vi "MIC_coMD.vi"() -> ()   [LabVIEW 2012]
doc: "SciScan 1.2 160622"
uses:
  GFG/GFGfpRefGet.vi
  GFG/GFGnumericGet.vi
  GFG/GFG library.lvlib
panel:
  out "Source VI":string
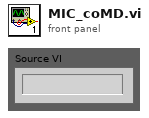
[diagram p1: front panel]
types:
  T1 = enum8{"Enabled", "Disabled", "Disabled and Grayed Out"}
  T2 = cluster{"WaveformChartRef":refnum<vi>, "DigitalRef":refnum<vi>, "ArrayRef":refnum<vi>, "TabControlRef":refnum<vi>, "EnumRef":refnum<vi>, "RingRef":refnum<vi>, "BooleanRef":refnum<vi>, "KnobRef":refnum<vi>, "SlideRef":refnum<vi>, "PathRef":refnum<vi>, "StringRef":refnum<vi>, "ComboBox":refnum<vi>, "WaveformGraphRef":refnum<vi>}
  T3 = enum16{"Left Button", "Center Button", "Right Button", "Window Close"}
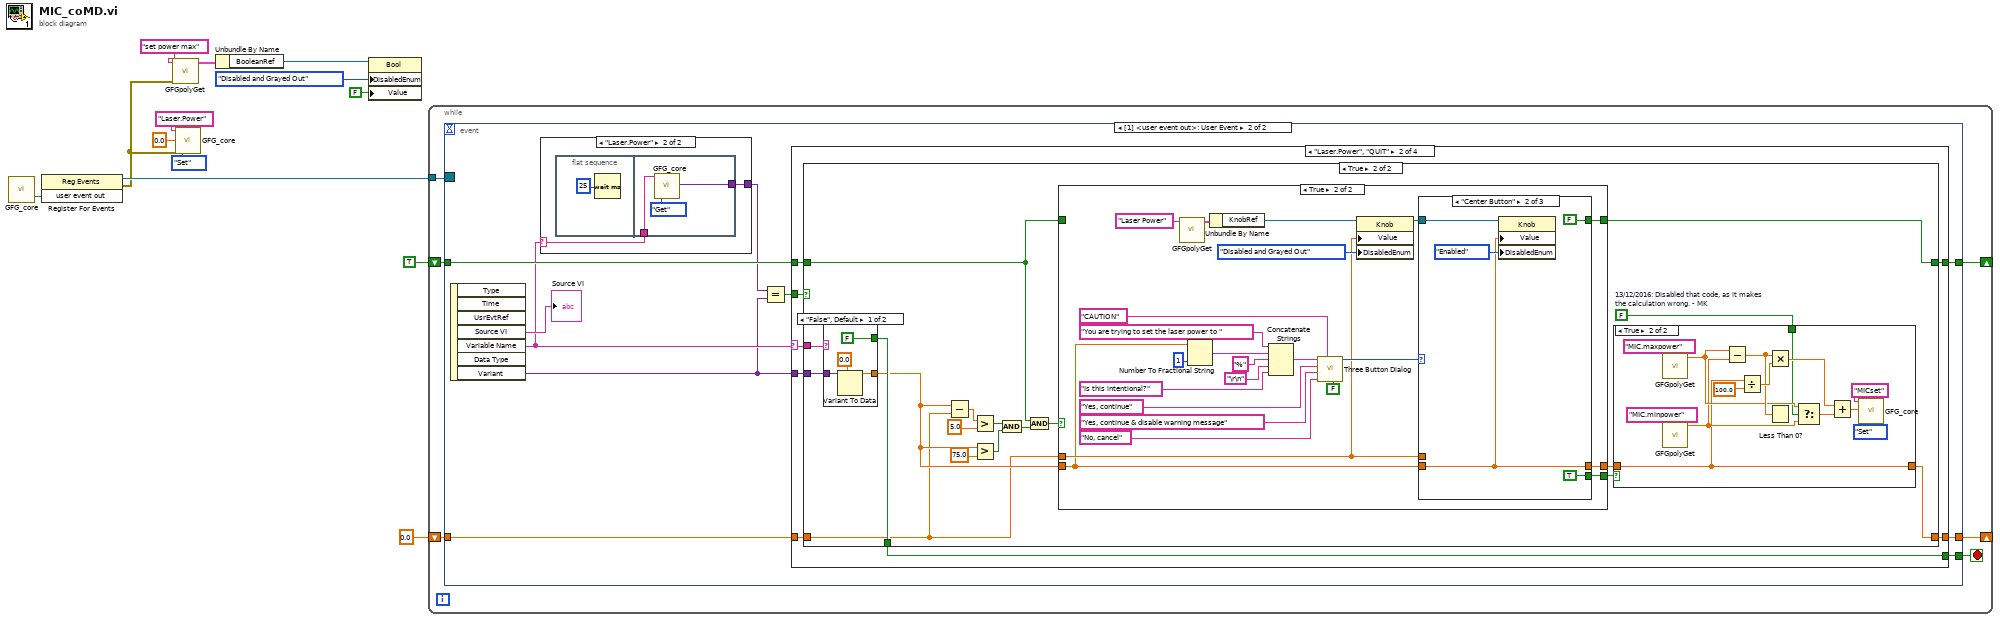
[diagram p0: block diagram]
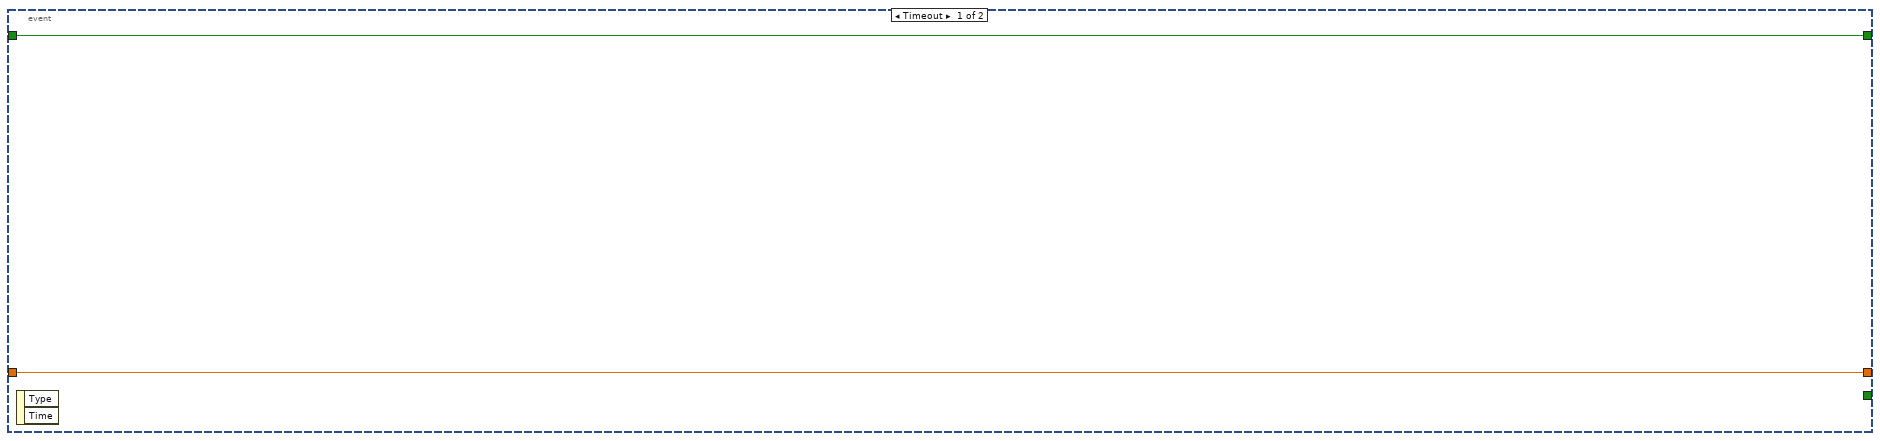
[diagram p2: hidden frame]
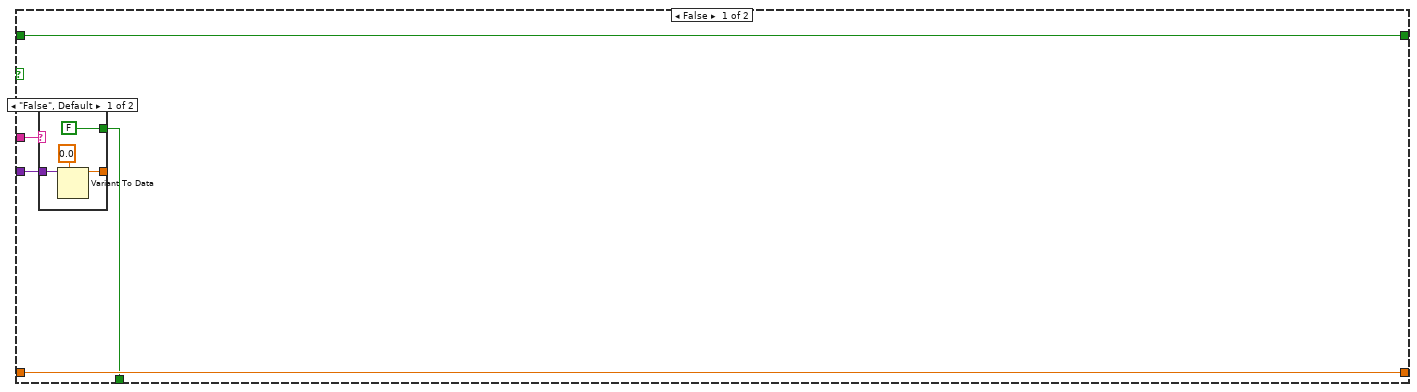
[diagram p5: hidden frame]
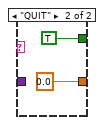
[diagram p6: hidden frame]
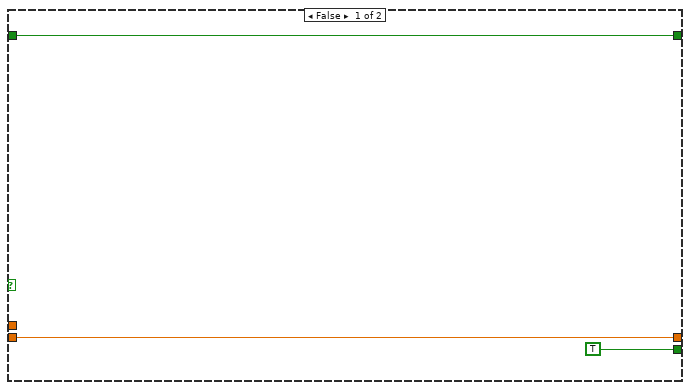
[diagram p8: hidden frame]
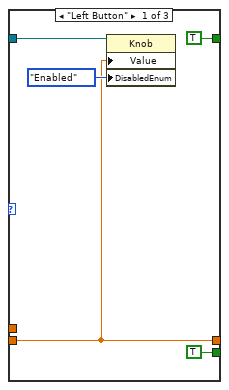
[diagram p9: hidden frame]
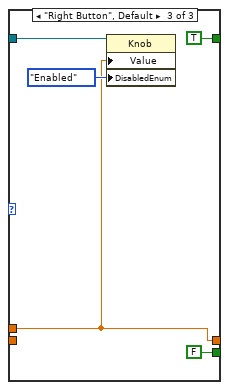
[diagram p10: hidden frame]
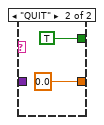
[diagram p11: hidden frame]
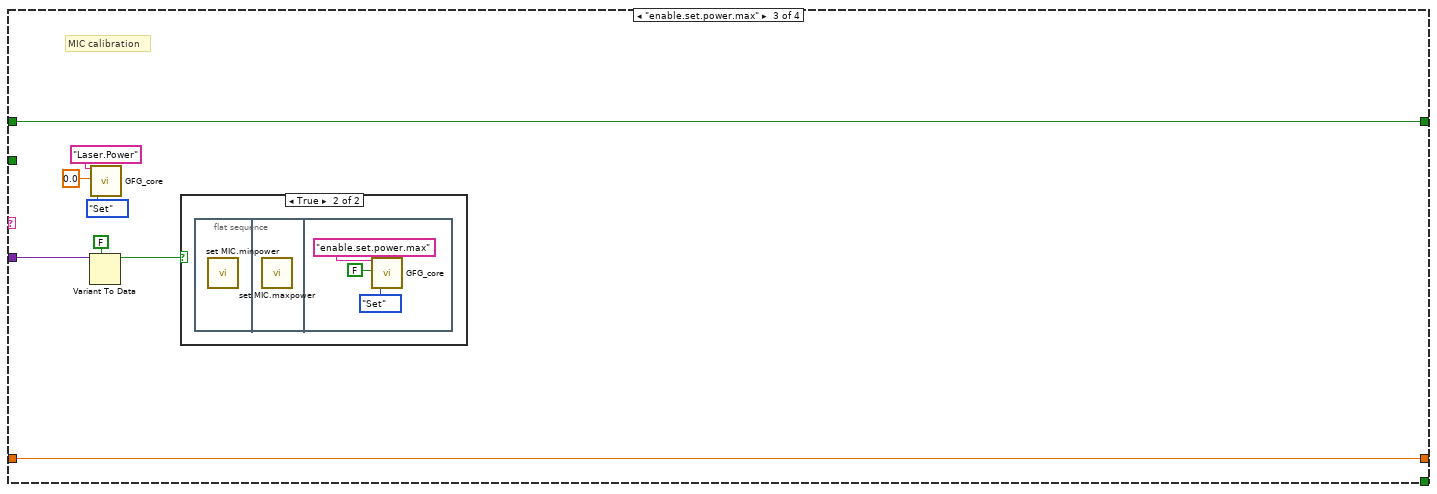
[diagram p12: hidden frame]
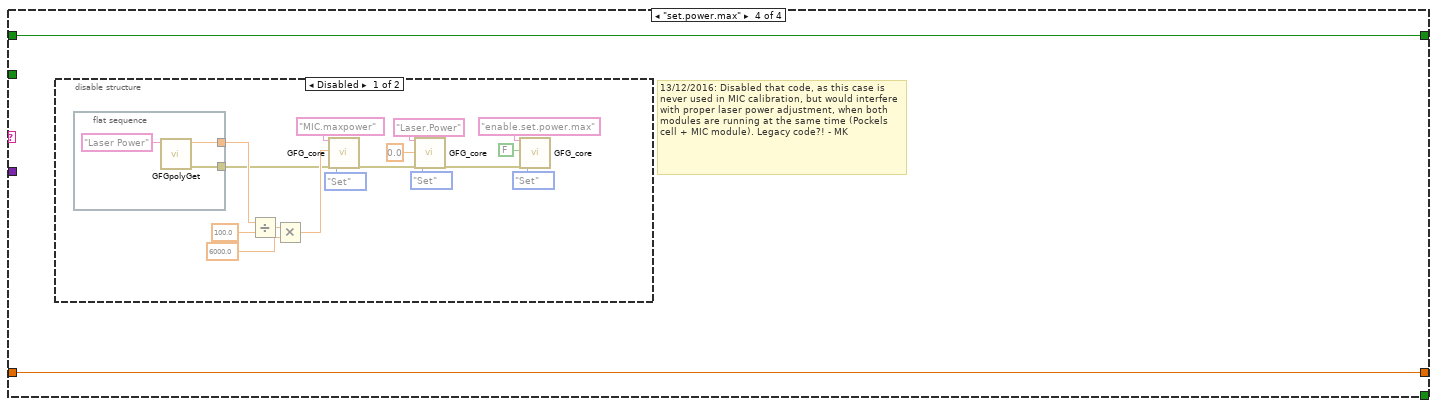
[diagram p14: hidden frame]
diagram:
  n1 = call "GFG_core.vi"() -> ("user event out"=w13:refnum<user-event>)  [unwired: 13 in, 6 out]
  n2 = register-events(w13) -> (reference out=w12:refnum<event-registration>, error out=w1:errorcluster)  [unwired: 2 in]
  n3 = call-poly "GFGpolyGet.vi"("error in (no error)"=w1, "Variable Name in"="set power max") -> ("output cluster"=w4:T2)  [unwired: 8 in, 1 out]
  n4 = call "GFG_core.vi"("Variable Name in"="Laser.Power", "Variant in"=0.0 ("Laser Power"), "error in (no error)"=w1, "Action"=enum16{"Init", "Set", "Get"}."Set") -> ()  [unwired: 9 in, 7 out]
  n5 = Unbundle By Name(w4) -> ("BooleanRef"=w5:refnum<vi>)
  n6 = property class="Bool"(reference=w5, "DisabledEnum"=T1."Disabled and Grayed Out" ("Disabled"), "Value"=FALSE) -> ()  [unwired: 1 in, 2 out]
  n7 = while {
    tunnel: w12 -> [w19]
    shift-right: [w17] -> _
    shift-left: 0.0 ("Laser Power") -> [w16]
    shift-right: [w15] -> _
    shift-left: TRUE -> [w14]
    stop <- w18 stop-if-true
    n8 = event shown="[1] <user event out>: User Event" {
      selector: w19 -> [_ _]
      dyn-events: _ -> [_ _]
      timeout: _ -> [_ _]
      tunnel: [_ w30] -> w18
      tunnel: [w21 w29] -> w17
      tunnel: w16 -> [w21 w28]
      tunnel: [w20 w27] -> w15
      tunnel: w14 -> [w20 w26]
      event Timeout {
        n9 = event-data() -> ()  [unwired: 1 in, 2 out]
      }
      event User Event {
        n10 = event-data() -> ("Source VI"=→"Source VI":string, "Variable Name"=w23:string, "Variant"=w22:variant)  [unwired: 1 in, 4 out]
        n11 = case shown="\"Laser.Power\"" w23 {
          selector: w23 -> [w32 w33]
          tunnel: [w32 w34] -> w25
          frame "False", Default {
          }
          frame "Laser.Power" {
            n12 = flat-sequence {
              tunnel: w33 -> [w37]
              tunnel: [w36] -> w34
              frame #0 {
                n13 = Wait (ms)(milliseconds to wait=u32 25) -> ()  [unwired: 1 out]
              }
              frame #1 {
                n14 = call "GFG_core.vi"("Variable Name in"=w37, "Action"=enum16{"Init", "Set", "Get"}."Get") -> ("Variant Out"=w36:variant)  [unwired: 11 in, 6 out]
              }
            }
          }
        }
        n15 = Equal?(x=w25, y=w22) -> (x = y?=w24:bool)
        n16 = case shown="\"Laser.Power\", \"QUIT\"" w23 {
          selector: w23 -> [_ w47 _ _]
          tunnel: w22 -> [_ w48 w142 _]
          tunnel: [_ w46 _ _] -> w30
          tunnel: [w40 w43 w147 w152] -> w29
          tunnel: w28 -> [w40 w42 w147 w152]
          tunnel: [w39 w45 w146 w151] -> w27
          tunnel: w26 -> [w39 w44 w146 w151]
          tunnel: w24 -> [_ w41 _ _]
          frame Default {
          }
          frame "Laser.Power", "QUIT" {
            n17 = case shown="True" w41 {
              tunnel: w48 -> [w51 w77]
              tunnel: w47 -> [w50 w76]
              tunnel: [w49 w75] -> w46
              tunnel: [w52 w72] -> w45
              tunnel: w44 -> [w52 w70]
              tunnel: [w53 w61] -> w43
              tunnel: w42 -> [w53 w66]
              frame False {
                n18 = case shown="\"False\", Default" w50 {
                  tunnel: w51 -> [w57 _]
                  tunnel: [w56 0.0 ("Laser Power")] -> _
                  tunnel: [FALSE TRUE] -> w49
                  frame "False", Default {
                    n19 = Variant To Data(type=0.0 ("Laser Power"), Variant=w57) -> (data=w56:dbl)  [unwired: 1 in, 1 out]
                  }
                  frame "QUIT" {
                  }
                }
              }
              frame True {
                w60 = FALSE  # 13/12/2016: Disabled that code, as it makes the calculation wrong. - MK
                n20 = case shown="\"False\", Default" w76 {
                  tunnel: w77 -> [w137 _]
                  tunnel: [w136 0.0 ("Laser Power")] -> w67
                  tunnel: [FALSE TRUE] -> w75
                  frame "False", Default {
                    n21 = Variant To Data(type=0.0 ("Laser Power"), Variant=w137) -> (data=w136:dbl)  [unwired: 1 in, 1 out]
                  }
                  frame "QUIT" {
                  }
                }
                n22 = Subtract(x=w67, y=w66) -> (x-y=w65:dbl)
                n23 = Greater?(x=w65, y=5.0) -> (0:w63:bool)
                n24 = Greater?(x=w67, y=75.0) -> (0:w74:bool)
                n25 = And(x=w63, y=w74) -> (x .and. y?=w68:bool)
                n26 = And(x=w70, y=w68) -> (x .and. y?=w71:bool)
                n27 = case shown="True" w71 {
                  tunnel: [TRUE w112] -> w62
                  tunnel: [w94 w111] -> w72
                  tunnel: w70 -> [w94 _]
                  tunnel: w66 -> [_ w101]
                  tunnel: w67 -> [w93 w96]
                  tunnel: [w93 w97] -> w69
                  frame False {
                  }
                  frame True {
                    n28 = call-poly "GFGpolyGet.vi"("Variable Name in"="Laser Power") -> ("output cluster"=w105:T2)  [unwired: 9 in, 1 out]
                    n29 = Number To Fractional String(number=w96, precision (6)=i16 1) -> (F-format string=w100:string)  [unwired: 2 in]
                    n30 = Unbundle By Name(w105) -> ("KnobRef"=w104:refnum<vi>)
                    n31 = Concatenate Strings("You are trying to set the laser power to " ("message"), w100, "%" ("string"), "\r\n", "Is this intentional?" ("string")) -> (w107:string)
                    n32 = call <vilib>:"Three Button Dialog.vi"("Allow user to close window? (TRUE)"=FALSE, "Window Title (\"\")"="CAUTION" ("Window Title (\"\")"), "Right Button Text (\"Cancel\")"="No, cancel" ("Right Button Text (\"Cancel\")"), "Center Button Text (\"No\")"="Yes, continue & disable warning message" ("Center Button Text (\"No\")"), "Left Button Text (\"Yes\")"="Yes, continue" ("Left Button Text (\"Yes\")"), "message"=w107) -> ("Which Button?"=w113:T3)  [unwired: 5 in]
                    n33 = property class="Knob"(reference=w104, "Value"=w101, "DisabledEnum"=T1."Disabled and Grayed Out" ("Disabled")) -> (reference out=w102:refnum<vi>)  [unwired: 1 in, 1 out]
                    n34 = case shown="\"Center Button\"" w113 {
                      tunnel: [TRUE TRUE FALSE] -> w112
                      tunnel: [TRUE FALSE TRUE] -> w111
                      tunnel: w102 -> [w120 w125 w130]
                      tunnel: w96 -> [w119 w124 _]
                      tunnel: w101 -> [_ _ w129]
                      tunnel: [w119 w124 w129] -> w97
                      frame "Left Button" {
                        n35 = property class="Knob"(reference=w120, "Value"=w119, "DisabledEnum"=T1."Enabled" ("Disabled")) -> ()  [unwired: 1 in, 2 out]
                      }
                      frame "Center Button" {
                        n36 = property class="Knob"(reference=w125, "Value"=w124, "DisabledEnum"=T1."Enabled" ("Disabled")) -> ()  [unwired: 1 in, 2 out]
                      }
                      frame "Right Button", Default {
                        n37 = property class="Knob"(reference=w130, "Value"=w129, "DisabledEnum"=T1."Enabled" ("Disabled")) -> ()  [unwired: 1 in, 2 out]
                      }
                    }
                  }
                }
                n38 = case shown="True" w62 {
                  tunnel: w69 -> [w78 w80]
                  tunnel: [w78 w80] -> w61
                  tunnel: w60 -> [_ w79]
                  frame False {
                  }
                  frame True {
                    n39 = call-poly "GFGpolyGet.vi"("Variable Name in"="MIC.maxpower") -> ("Numeric"=w86:dbl)  [unwired: 8 in, 2 out]
                    n40 = call-poly "GFGpolyGet.vi"("Variable Name in"="MIC.minpower") -> ("Numeric"=w83:dbl)  [unwired: 8 in, 2 out]
                    n41 = Subtract(x=w86, y=w83) -> (x-y=w87:dbl)
                    n42 = Divide(x=w80, y=100.0 ("x")) -> (x/y=w92:dbl)
                    n43 = Multiply(x=w87, y=w92) -> (x*y=w90:dbl)
                    n44 = Less Than 0?(x=w87) -> ()  [unwired: 1 out]
                    n45 = Select(t=w86, s=w79, f=w83) -> (s? t:f=w84:dbl)
                    n46 = Add(x=w90, y=w84) -> (x+y=w85:dbl)
                    n47 = call "GFG_core.vi"("Variable Name in"="MICset", "Variant in"=w85, "Action"=enum16{"Init", "Set", "Get"}."Set") -> ()  [unwired: 10 in, 7 out]
                  }
                }
              }
            }
          }
          frame "enable.set.power.max" {
            # "MIC calibration"
            n48 = Variant To Data(type=FALSE, Variant=w142) -> (data=w140:bool)  [unwired: 1 in, 1 out]
            n49 = call "GFG_core.vi"("Variable Name in"="Laser.Power", "Variant in"=0.0 ("Laser Power"), "Action"=enum16{"Init", "Set", "Get"}."Set") -> ()  [unwired: 10 in, 7 out]
            n50 = case shown="True" w140 {
              frame False {
              }
              frame True {
                n51 = flat-sequence {
                  frame #0 {
                    n52 = call "set MIC.minpower.vi"() -> ()  [unwired: 12 in]
                  }
                  frame #1 {
                    n53 = call "set MIC.maxpower.vi"() -> ()  [unwired: 12 in]
                  }
                  frame #2 {
                    n54 = call "GFG_core.vi"("Variable Name in"="enable.set.power.max", "Variant in"=FALSE, "Action"=enum16{"Init", "Set", "Get"}."Set") -> ()  [unwired: 10 in, 7 out]
                  }
                }
              }
            }
          }
          frame "set.power.max" {
            # "13/12/2016: Disabled that code, as this case is never used in MIC calibration, but would interfere with proper laser power adjustment, when both modules are running at the same time (Pockels cell + MIC module). Legacy code?! - MK"
            n55 = disable-structure shown="Disabled" {
              frame Disabled {
                n56 = flat-sequence {
                  tunnel: [w170] -> w165
                  tunnel: [w169] -> w163
                  frame #0 {
                    n57 = call-poly "GFGpolyGet.vi"("Variable Name in"="Laser Power") -> ("error out"=w169:errorcluster, "Numeric"=w170:dbl)  [unwired: 8 in, 1 out]
                  }
                }
                n58 = Divide(x=w165, y=100.0 ("x")) -> (x/y=w157:dbl)
                n59 = Multiply(x=w157, y=6000.0 ("Laser Power")) -> (x*y=w164:dbl)
                n60 = call "GFG_core.vi"("Variable Name in"="MIC.maxpower", "Variant in"=w164, "error in (no error)"=w163, "Action"=enum16{"Init", "Set", "Get"}."Set") -> ("error out"=w162:errorcluster)  [unwired: 9 in, 6 out]
                n61 = call "GFG_core.vi"("Variable Name in"="Laser.Power", "Variant in"=0.0 ("Laser Power"), "error in (no error)"=w162, "Action"=enum16{"Init", "Set", "Get"}."Set") -> ("error out"=w159:errorcluster)  [unwired: 9 in, 6 out]
                n62 = call "GFG_core.vi"("Variable Name in"="enable.set.power.max", "Variant in"=FALSE, "error in (no error)"=w159, "Action"=enum16{"Init", "Set", "Get"}."Set") -> ()  [unwired: 9 in, 7 out]
              }
              frame Enabled {
              }
            }
          }
        }
      }
    }
  }
